vi "SetDataFormat.vi"(8 "Error In":errorcluster, 10 "Data Format":T1, 11 "Keithley 6485 In":refnum<visa-resource-name>) -> (0 "Error Out":errorcluster, 3 "Keithley 6485 Out":refnum<visa-resource-name>)   [LabVIEW 2012, in "Keithley-6485.lvlib"]
uses:
  Keithley-6485.lvlib
  Controls/DataFormat.ctl
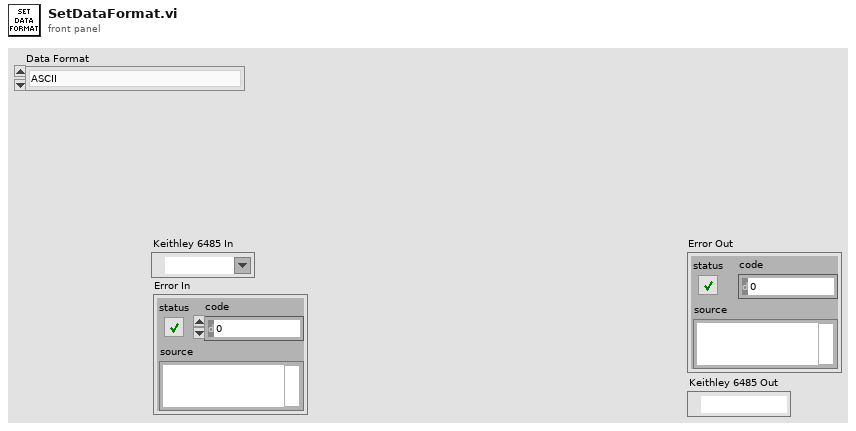
[diagram p1: front panel]
types:
  T1 = typedef "Keithley-6485.lvlib/DataFormat.ctl" = enum16{"ASCII", "Real", "32", "Sreal"}
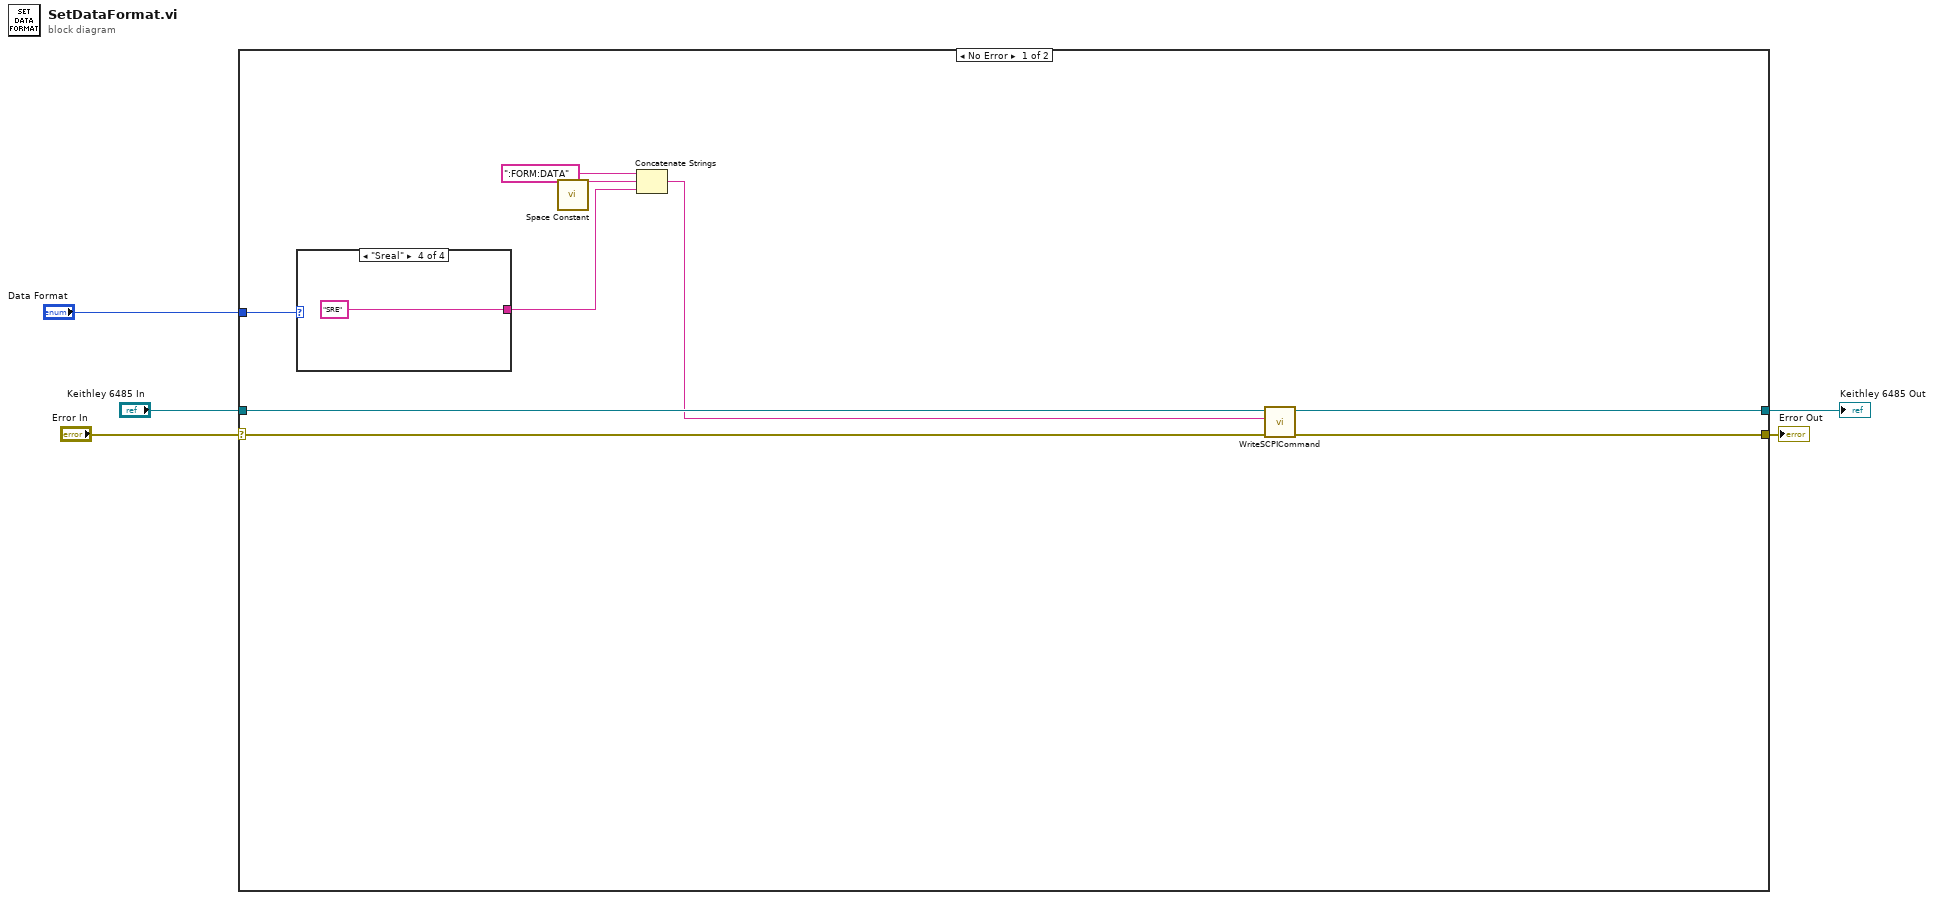
[diagram p0: block diagram]
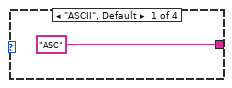
[diagram p2: hidden frame]
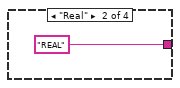
[diagram p3: hidden frame]
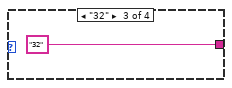
[diagram p4: hidden frame]
diagram:
  n1 = case shown="No Error" "Error In" {
    selector: "Error In" -> [w9 w19]
    tunnel: "Keithley 6485 In" -> [w8 w20]
    tunnel: [w10 w19] -> w3
    tunnel: [w11 w20] -> w2
    tunnel: "Data Format" -> [w6 _]
    frame No Error {
      n2 = case shown="\"Sreal\"" w6 {
        tunnel: ["ASC" "REAL" "32" "SRE"] -> w12
        frame "ASCII", Default {
        }
        frame "Real" {
        }
        frame "32" {
        }
        frame "Sreal" {
        }
      }
      n3 = call <vilib>:"Space Constant.vi"() -> ("String"=w13:string)
      n4 = Concatenate Strings(":FORM:DATA", w13, w12) -> (w7:string)
      n5 = call "WriteSCPICommand.vi"("Error In"=w9, "SCPI Command"=w7, "Keithley 6482 In"=w8) -> ("Error Out"=w10:errorcluster, "Keithley 6482 Out"=w11:refnum<visa-resource-name>)  [unwired: 7 in]
    }
    frame Error {
    }
  }
  "Error Out" <- w3
  "Keithley 6485 Out" <- w2
